vi "send and receive pmt data.vi"(7 "data (byte array)":u8[](array[numeric]), 8 "error in (no error)":errorcluster, 9 "data (byte)":u8, 10 "Command":T1, 11 "VISA resource":refnum<visa-resource-name>) -> (0 "error out":errorcluster, 1 "all data received":bool, 2 "data out":u8[](array[numeric]), 3 "visa out":refnum<visa-resource-name>)   [LabVIEW 2017]
uses:
  pmt demultiplexer command set.ctl
  <vilib>/Instr/_visa.llb/VISA Flush IO Buffer Mask.ctl
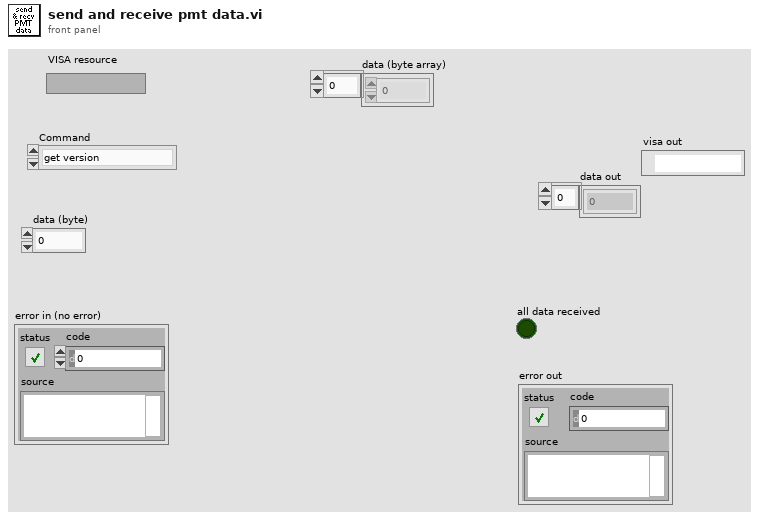
[diagram p1: front panel]
types:
  T1 = typedef "pmt demultiplexer command set.ctl" = enum8{"get version", "set outputs", "set pll", "get histogram", "set passthrough", "set pmt veto", "reset pll", "set test inputs", "get error"}
  T2 = typedef "VISA Flush IO Buffer Mask.ctl" = u16
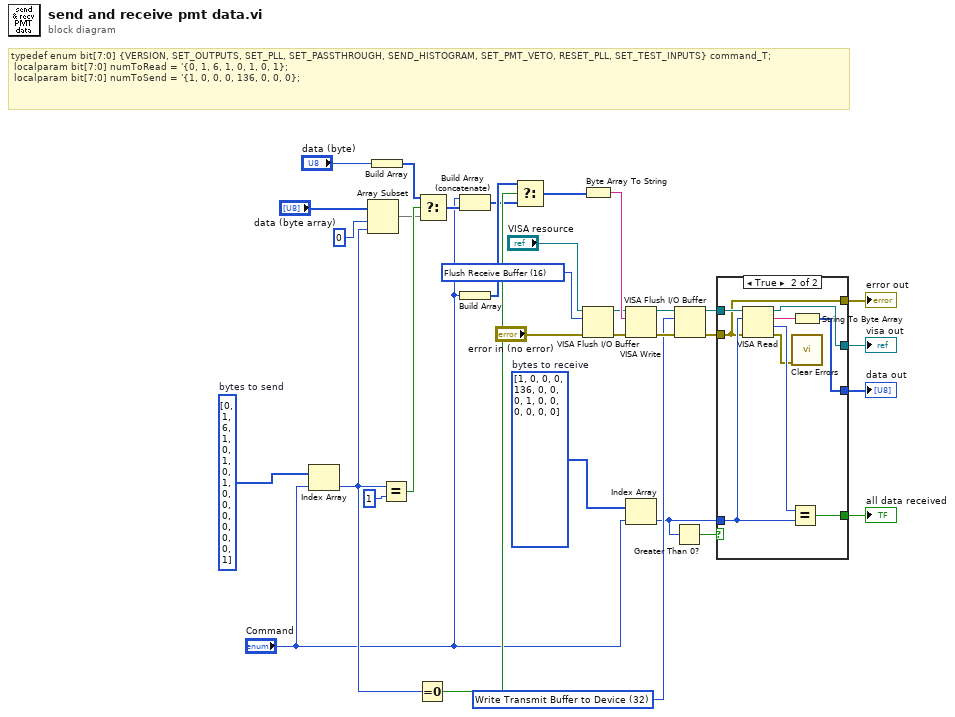
[diagram p0: block diagram]
diagram:
  w1 = T2 16 items=["Flush Receive Buffer"=16, "Write Transmit Buffer to Device"=32, "Flush Receive Buffer (No I/O)"=64, "Flush Transmit Buffer"=128] ("Mask")
  w16 = T2 32 items=["Flush Receive Buffer"=16, "Write Transmit Buffer to Device"=32, "Flush Receive Buffer (No I/O)"=64, "Flush Transmit Buffer"=128] ("Mask")
  w14 = i32[] [1, 0, 0, 0, 136, 0, 0, 0, 1, 0, 0, 0, 0, 0, 0]  # bytes to receive
  w33 = i32[] [0, 1, 6, 1, 0, 1, 0, 1, 0, 0, 0, 0, 0, 0, 1]  # bytes to send
  # "typedef enum bit[7:0] {VERSION, SET_OUTPUTS, SET_PLL, SET_PASSTHROUGH, SEND_HISTOGRAM, SET_PMT_VETO, RESET_PLL, SET_TEST_INPUTS} command_T; \n\tlocalparam bit[7:0] numToRead = '{0, 1, 6, 1, 0, 1, 0, 1};\n\tlocalparam bit[7:0] numToSend = '{1, 0, 0, 0, 136, 0, 0, 0};"
  n1 = Index Array(array=w33, index="Command") -> (element=w23:i32)
  n2 = Array Subset(array="data (byte array)", index=0, length=w23) -> (w22:u8[])
  n3 = Build Array("data (byte)") -> (w27:u8[])
  n4 = Equal?(x=w23, y=1) -> (x = y?=w29:bool)
  n5 = Equal To 0?(x=w23) -> (x = 0?=w32:bool)
  n6 = Select(t=w27, s=w29, f=w22) -> (s? t:f=w26:u8[])
  n7 = Build Array (concatenate)("Command", w26) -> (w21:u8[])
  n8 = Build Array("Command") -> (w31:T1[])
  n9 = Select(t=w31, s=w32, f=w21) -> (s? t:f=w19:u8[])
  n10 = Byte Array To String(unsigned byte array=w19) -> (string=w20:string)
  n11 = VISA Flush I/O Buffer(VISA resource name="VISA resource", mask (16)=w1, error in (no error)="error in (no error)") -> (VISA resource name out=w2:refnum<visa-resource-name>, error out=w3:errorcluster)
  n12 = VISA Write(VISA resource name=w2, write buffer=w20, error in (no error)=w3) -> (VISA resource name out=w18:refnum<visa-resource-name>, error out=w17:errorcluster)  [unwired: 1 out]
  n13 = Index Array(array=w14, index="Command") -> (element=w12:i32)
  n14 = Greater Than 0?(x=w12) -> (x > 0?=w13:bool)
  n15 = VISA Flush I/O Buffer(VISA resource name=w18, mask (16)=w16, error in (no error)=w17) -> (VISA resource name out=w10:refnum<visa-resource-name>, error out=w11:errorcluster)
  n16 = case shown="True" w13 {
    tunnel: w12 -> [_ w42]
    tunnel: w11 -> [w35 w40]
    tunnel: w10 -> [w34 w44]
    tunnel: [w35 w40] -> w6
    tunnel: [_ w39] -> w9
    tunnel: [w34 w38] -> w7
    tunnel: [_ w36] -> w8
    frame False {
    }
    frame True {
      n17 = VISA Read(VISA resource name=w44, byte count=w42, error in (no error)=w40) -> (VISA resource name out=w38:refnum<visa-resource-name>, read buffer=w37:string, return count=w43:u32, error out=w41:errorcluster)
      n18 = Equal?(x=w43, y=w42) -> (x = y?=w39:bool)
      n19 = String To Byte Array(string=w37) -> (unsigned byte array=w36:u8[])
      n20 = call <vilib>:"Clear Errors.vi"("error in (no error)"=w41) -> ()  [unwired: 5 in, 2 out]
    }
  }
  "all data received" <- w9
  "data out" <- w8
  "visa out" <- w7
  "error out" <- w6
